vi "Facade Custom Time Display.vi"(0 "Data In":T4, 2 "Display State In":T2, 3 "Container State":T3) -> (6 "Data Out":T4, 7 "Display State Out":T2, 8 "Action":T1)   [LabVIEW 2016, in "XControl Custom Time Display.xctl"]
uses:
  XControl Custom Time Display.xctl
  Data Custom Time Display.ctl
  <vilib>/_xctls/Container State.ctl
  State Custom Time Display.ctl
  <vilib>/_xctls/Action.ctl
  <vilib>/_xctls/XControlSupport.lvlib
panel:
  out "String":string caption="Timer"
  # "1. Drop the controls that make up the appearance\nof the XControl here.\n\n2. Resize the window to fit the controls\n\n3. If the XControl is of fixed size,  make the \n window not resizable from VI Properties->Window Appearance.\n\n4. If you want the controls to automatically size when the XControl sizes, check  \"Scale all objects on front panel when window resizes\" in File->VI Properties->Window Size page.\n\n5. Show the block diagram and handle events for the controls on this panel."
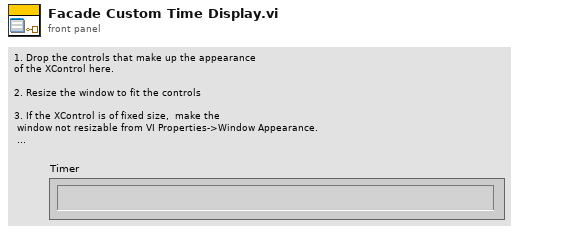
[diagram p1: front panel]
types:
  T1 = typedef "XControlSupport.lvlib/Action.ctl" = cluster{"Data Changed?":bool, "State Changed?":bool, "Action Name":string}
  T2 = typedef "XControl Custom Time Display.xctl/State Custom Time Display.ctl" = cluster{"Caption Mine":string}
  T3 = typedef "XControlSupport.lvlib/Container State.ctl" = cluster{"Indicator?":bool, "Run Mode?":bool, " Refnum":refnum<vi>}
  T4 = typedef "XControl Custom Time Display.xctl/Data Custom Time Display.ctl" = dbl
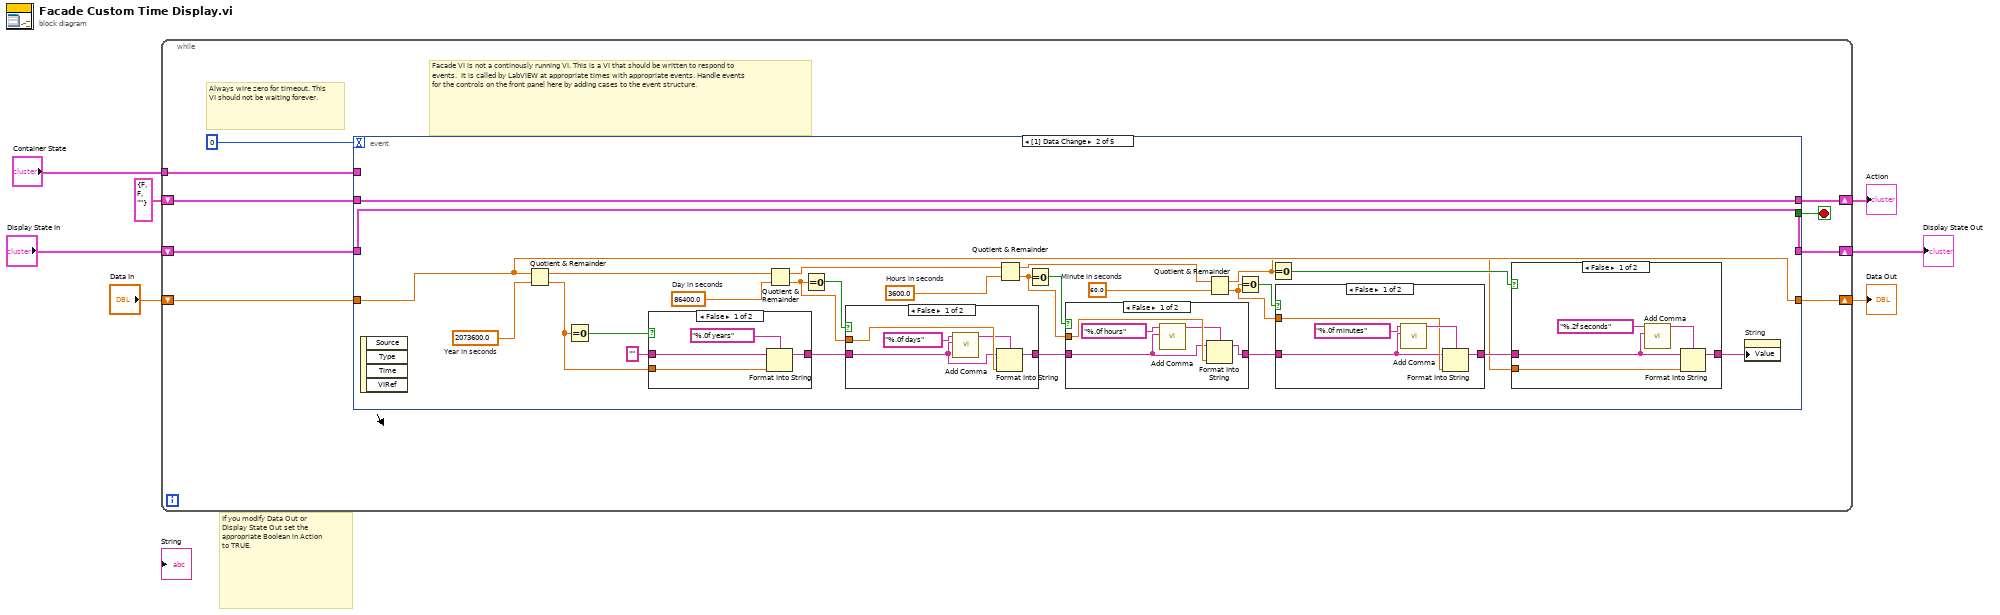
[diagram p0: block diagram]
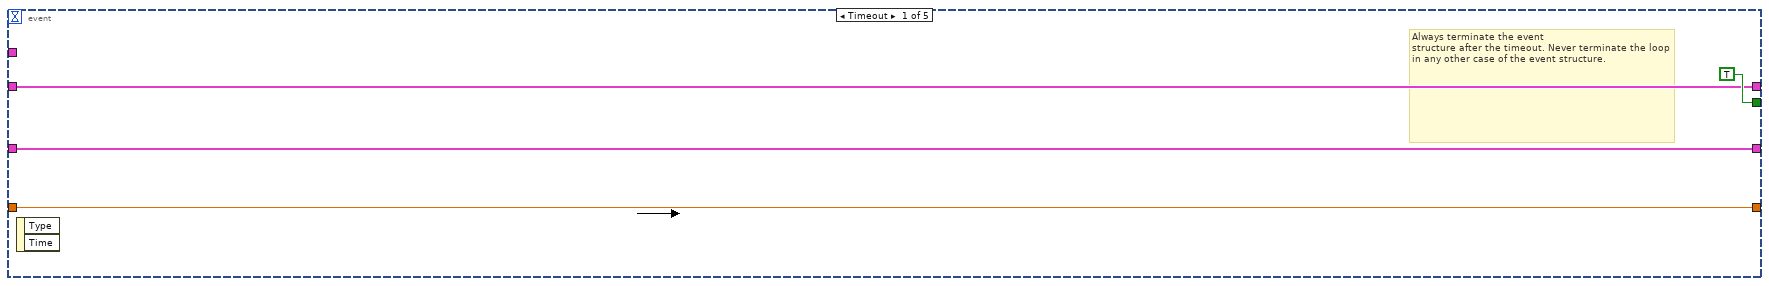
[diagram p2: hidden frame]
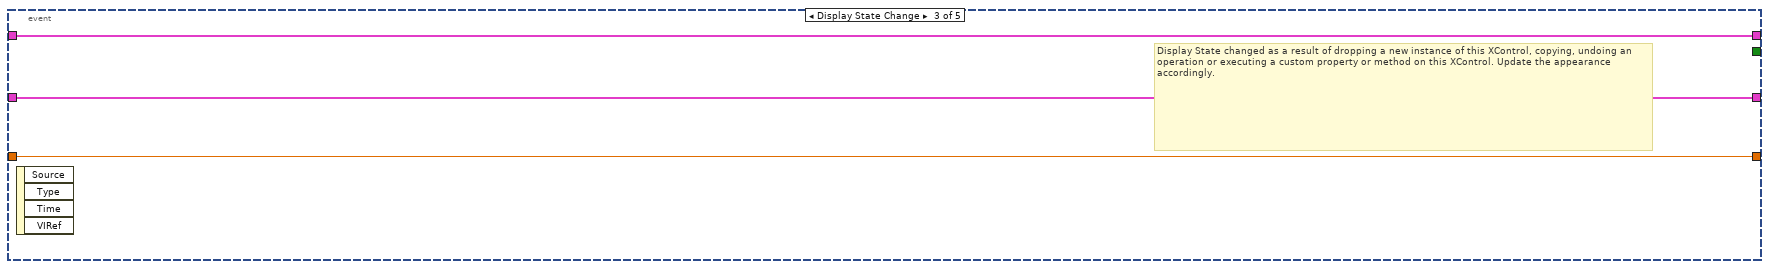
[diagram p8: hidden frame]
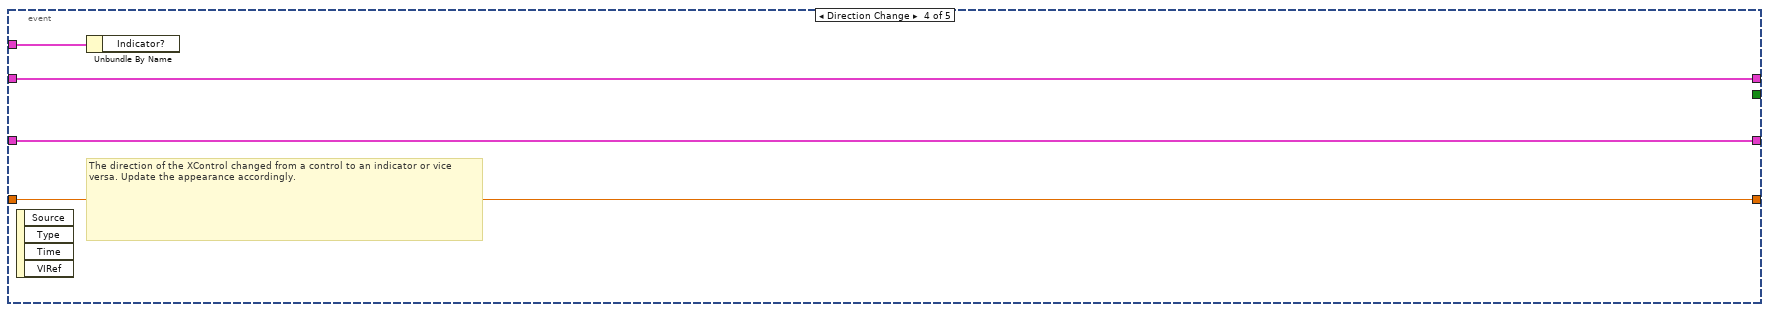
[diagram p9: hidden frame]
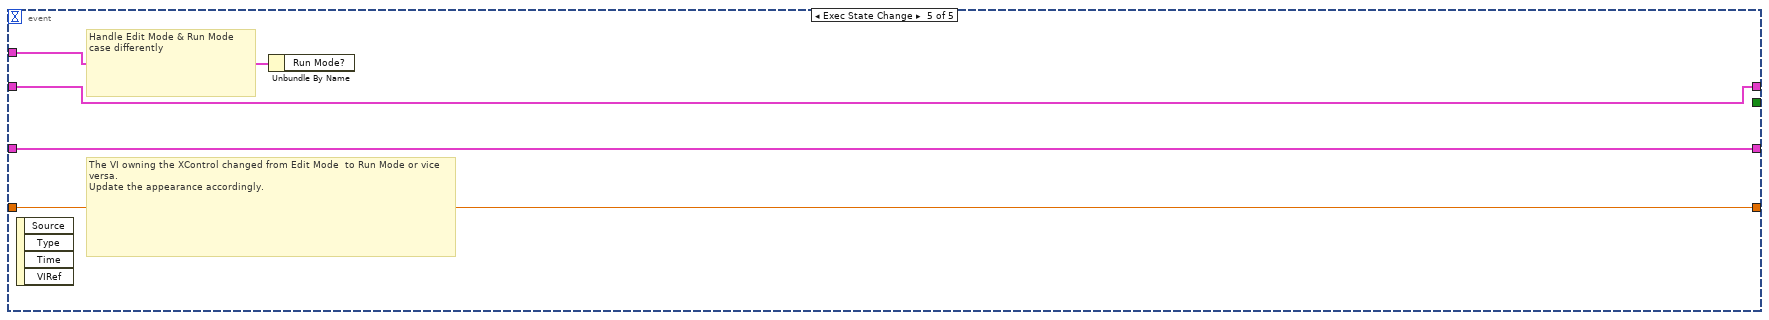
[diagram p10: hidden frame]
diagram:
  # "If you modify Data Out or\nDisplay State Out set the\nappropriate Boolean in Action\nto TRUE."
  n1 = while {
    shift-right: [w15] -> w4
    shift-left: "Display State In" -> [w16]
    tunnel: "Container State" -> [w12]
    shift-right: [w10] -> w7
    shift-left: "Data In" -> [w11]
    shift-right: [w8] -> w2
    shift-left: T1 {"Data Changed?"=FALSE, "State Changed?"=FALSE, "Action Name"=""} ("Action") -> [w9]
    stop <- w14 stop-if-true
    # "Facade VI is not a continously running VI. This is a VI that should be written to respond to events.  It is called by LabVIEW at appropriate times with appropriate events. Handle events for the controls on the front panel here by adding cases to the event structure."
    # "Always wire zero for timeout. This\nVI should not be waiting forever."
    n2 = event shown="[1] Data Change" {
      selector: _ -> [_ _ _ _ _]
      dyn-events: _ -> [_ _ _ _ _]
      timeout: 0 -> [_ _ _ _ _]
      tunnel: w16 -> [w18 w45 w78 w81 w85]
      tunnel: [w18 w45 w78 w81 w85] -> w15
      tunnel: [TRUE _ _ _ _] -> w14
      tunnel: w12 -> [_ _ _ w82 w86]
      tunnel: w11 -> [w17 w44 w77 w80 w84]
      tunnel: [w17 w44 w77 w80 w84] -> w10
      tunnel: [w19 w46 w76 w79 w83] -> w8
      tunnel: w9 -> [w19 w46 w76 w79 w83]
      event Timeout {
        # "Always terminate the event\nstructure after the timeout. Never terminate the loop in any other case of the event structure."
        n3 = event-data() -> ()  [unwired: 1 in, 2 out]
      }
      event Data Change {
        w42 = T4 86400.0  # Day in seconds
        w40 = T4 60.0  # Minute in seconds
        w41 = T4 3600.0  # Hours in seconds
        w43 = T4 2073600.0  # Year in seconds
        n4 = event-data() -> ()  [unwired: 1 in, 4 out]
        n5 = Quotient & Remainder(x=w44, y=w43) -> (x-y*floor(x/y)=w30:T4, floor(x/y)=w31:T4)
        n6 = Equal To 0?(x=w31) -> (x = 0?=w39:bool)
        n7 = case shown="False" w39 {
          tunnel: "" -> [w74 w75]
          tunnel: [w71 w75] -> w32
          tunnel: w31 -> [w73 _]
          frame False {
            n8 = Format Into String(format string="%.0f years", initial string=w74, w73) -> (resulting string=w71:string)  [unwired: 1 in, 1 out]
          }
          frame True {
          }
        }
        n9 = Quotient & Remainder(x=w30, y=w42) -> (x-y*floor(x/y)=w28:T4, floor(x/y)=w29:T4)
        n10 = Equal To 0?(x=w29) -> (x = 0?=w38:bool)
        n11 = case shown="False" w38 {
          tunnel: [w68 w70] -> w33
          tunnel: w32 -> [w65 w70]
          tunnel: w29 -> [w69 _]
          frame False {
            n12 = call "Add Comma.vi"("Previous String"=w65, "format string in"="%.0f days" ("format string")) -> ("format string out"=w66:string)  [unwired: 9 in]
            n13 = Format Into String(format string=w66, initial string=w65, w69) -> (resulting string=w68:string)  [unwired: 1 in, 1 out]
          }
          frame True {
          }
        }
        n14 = Quotient & Remainder(x=w28, y=w41) -> (x-y*floor(x/y)=w26:T4, floor(x/y)=w27:T4)
        n15 = Equal To 0?(x=w27) -> (x = 0?=w37:bool)
        n16 = case shown="False" w37 {
          tunnel: [w62 w64] -> w34
          tunnel: w33 -> [w59 w64]
          tunnel: w27 -> [w63 _]
          frame False {
            n17 = call "Add Comma.vi"("Previous String"=w59, "format string in"="%.0f hours" ("format string")) -> ("format string out"=w60:string)  [unwired: 9 in]
            n18 = Format Into String(format string=w60, initial string=w59, w63) -> (resulting string=w62:string)  [unwired: 1 in, 1 out]
          }
          frame True {
          }
        }
        n19 = Quotient & Remainder(x=w26, y=w40) -> (x-y*floor(x/y)=w21:T4, floor(x/y)=w25:T4)
        n20 = Equal To 0?(x=w25) -> (x = 0?=w36:bool)
        n21 = Equal To 0?(x=w21) -> (x = 0?=w24:bool)
        n22 = case shown="False" w36 {
          tunnel: [w57 w58] -> w22
          tunnel: w34 -> [w53 w58]
          tunnel: w25 -> [w54 _]
          frame False {
            n23 = call "Add Comma.vi"("Previous String"=w53, "format string in"="%.0f minutes") -> ("format string out"=w56:string)  [unwired: 9 in]
            n24 = Format Into String(format string=w56, initial string=w53, w54) -> (resulting string=w57:string)  [unwired: 1 in, 1 out]
          }
          frame True {
          }
        }
        n25 = case shown="False" w24 {
          tunnel: w22 -> [w49 w52]
          tunnel: [w48 w52] -> w23
          tunnel: w21 -> [w47 _]
          frame False {
            n26 = call "Add Comma.vi"("Previous String"=w49, "format string in"="%.2f seconds") -> ("format string out"=w51:string)  [unwired: 9 in]
            n27 = Format Into String(format string=w51, initial string=w49, w47) -> (resulting string=w48:string)  [unwired: 1 in, 1 out]
          }
          frame True {
          }
        }
        n28 = property on="String" class="Str"("Value"=w23) -> ()  [unwired: 2 in, 2 out]
      }
      event Display State Change {
        # "Display State changed as a result of dropping a new instance of this XControl, copying, undoing an operation or executing a custom property or method on this XControl. Update the appearance accordingly."
        n29 = event-data() -> ()  [unwired: 1 in, 4 out]
      }
      event Direction Change {
        # "The direction of the XControl changed from a control to an indicator or vice versa. Update the appearance accordingly."
        n30 = event-data() -> ()  [unwired: 1 in, 4 out]
        n31 = Unbundle By Name(w82) -> ()  [unwired: 1 out]
      }
      event Exec State Change {
        # "The VI owning the XControl changed from Edit Mode  to Run Mode or vice versa.\nUpdate the appearance accordingly."
        # "Handle Edit Mode & Run Mode\ncase differently"
        n32 = event-data() -> ()  [unwired: 1 in, 4 out]
        n33 = Unbundle By Name(w86) -> ()  [unwired: 1 out]
      }
    }
  }
  "Display State Out" <- w4
  "Data Out" <- w7
  "Action" <- w2
